vi "IntuitiveSteering_sineGenerator.vi"(9 "Phase Shift":dbl, 10 "Forward Time":dbl, 11 "Input":dbl) -> (3 "Fin Position":dbl[](array[numeric]))   [LabVIEW 2013]
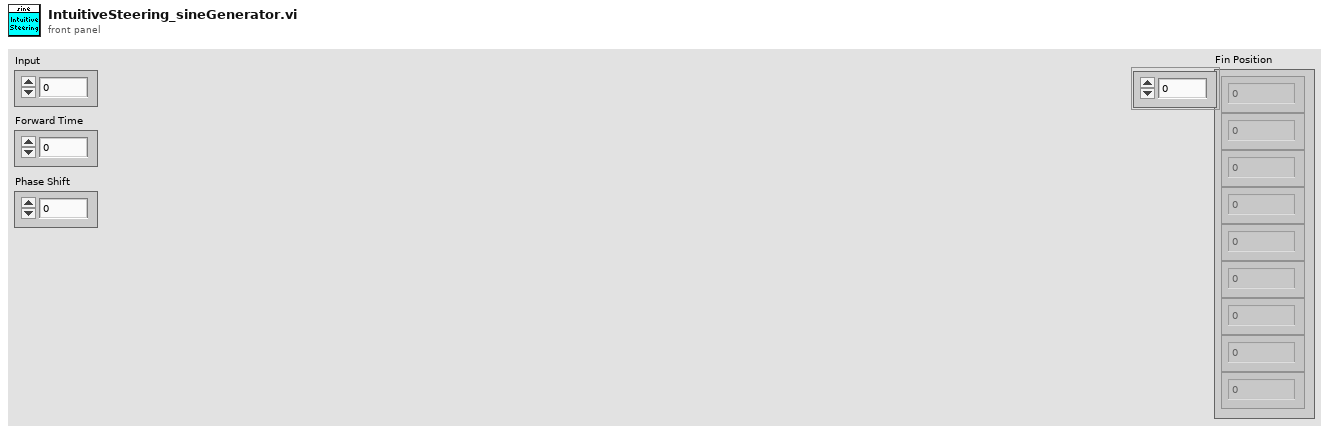
[diagram p1: front panel]
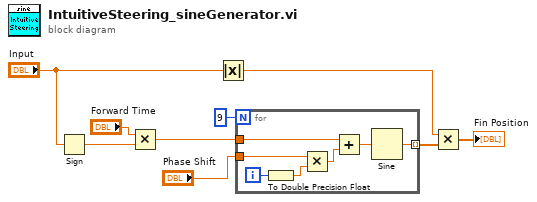
[diagram p0: block diagram]
diagram:
  n1 = Sign(1:"Input") -> (0:w3:dbl)
  n2 = Multiply(x="Forward Time", y=w3) -> (x*y=w2:dbl)
  n3 = Absolute Value(x="Input") -> (abs(x)=w7:dbl)
  n4 = for {
    N: 9 -> [_]
    tunnel: "Phase Shift" -> [w16]
    tunnel: w2 -> [w12]
    tunnel: [w10] -> w6 mode=indexing
    i -> [w15]
    n5 = To Double Precision Float(number=w15) -> (double precision float=w14:dbl)
    n6 = Multiply(x=w16, y=w14) -> (x*y=w13:dbl)
    n7 = Add(x=w12, y=w13) -> (x+y=w11:dbl)
    n8 = Sine(x=w11) -> (sin(x)=w10:dbl)
  }
  n9 = Multiply(x=w7, y=w6) -> (x*y=→"Fin Position":dbl[])
